vi "MemberAttendance Factory.vi"(8 "error in (no error)":errorcluster, 10 "2D Data":string[][](array[string]), 11 "ExcelReader in":refnum<class "ExcelReader.lvclass">) -> (0 "error out":errorcluster, 2 "MemberAttendance":refnum<class "MemberAttendance.lvclass">[](array[class]), 3 "ExcelReader out":refnum<class "ExcelReader.lvclass">)   [LabVIEW 2015, in "Admin_Actor.lvlib" / "ExcelReader.lvclass"]
uses:
  ExcelReader.lvclass
  MemberAttendance/MemberAttendance.lvclass
  g_variable/g_Excel Attributes.vi
  Database/Date_Excel/ExceelDate.lvclass
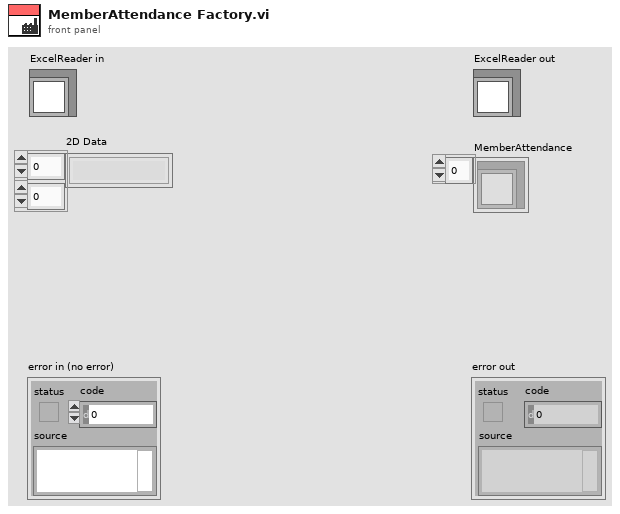
[diagram p1: front panel]
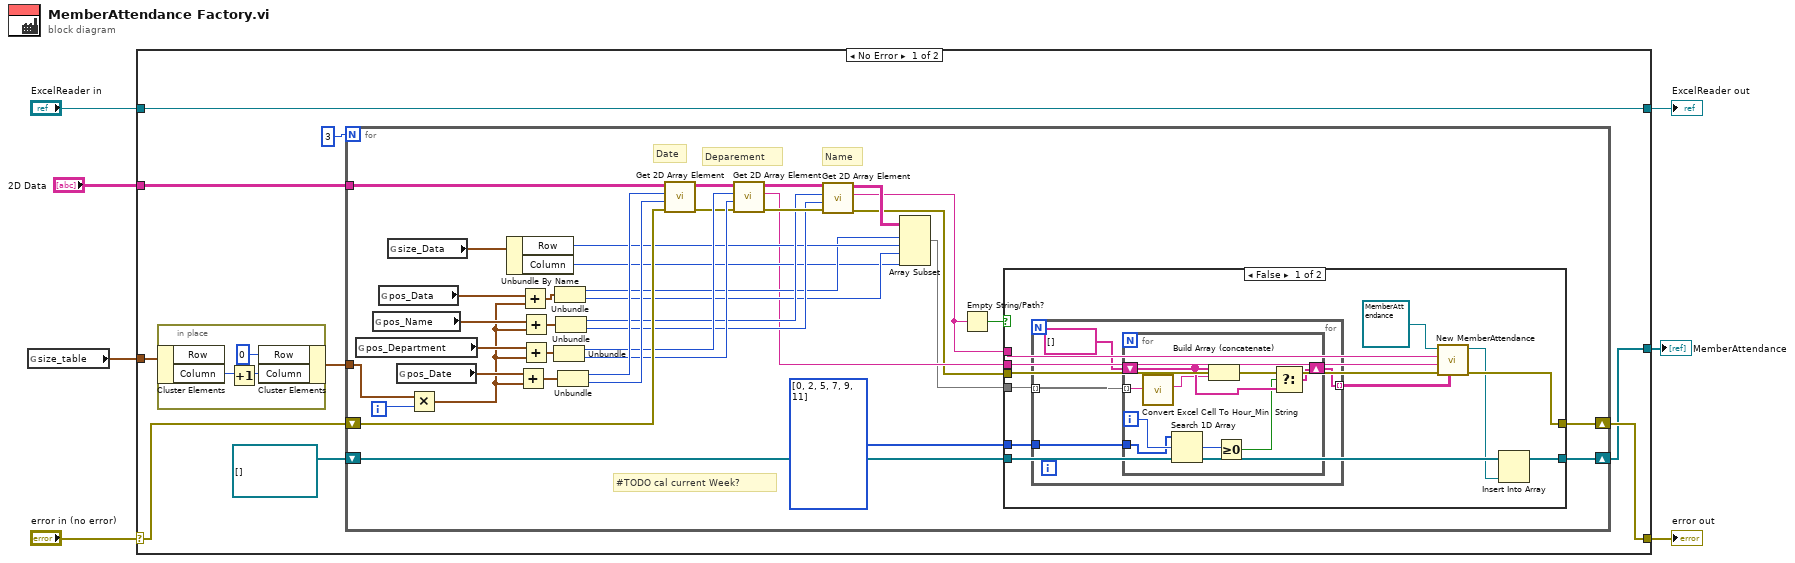
[diagram p0: block diagram]
diagram:
  n1 = global read "g_Excel Attributes.vi" "size_table"() -> (w2:cluster{"Row":i32, "Column":i32})
  n2 = case shown="No Error" "error in (no error)" {
    selector: "error in (no error)" -> [w13 w85]
    tunnel: [w12 w85] -> w6
    tunnel: [w16 w84] -> w4
    tunnel: "ExcelReader in" -> [w16 w84]
    tunnel: "2D Data" -> [w14 _]
    tunnel: w2 -> [w9 _]
    tunnel: [w10 _] -> w1
    frame No Error {
      n3 = in-place {
        n4 = in-place-cluster #1(w9) -> ("Column"=w19:i32)  [unwired: 1 out]
        n5 = Increment(x=w19) -> (x+1=w18:i32)
        n6 = in-place-cluster #1("Row"=0, "Column"=w18) -> (w8:cluster{"Row":i32, "Column":i32})
      }
      n7 = for {
        N: 3 -> [_]
        tunnel: w8 -> [w57]
        tunnel: w14 -> [w49]
        shift-right: [w25] -> w12
        shift-left: w13 -> [w51]
        shift-right: [w21] -> w10
        shift-left: refnum<class "MemberAttendance.lvclass">[] [] ("Array") -> [w24]
        i -> [w56]
        # "#TODO cal current Week?"
        # "Name"
        # "Deparement"
        # "Date"
        n8 = global read "g_Excel Attributes.vi" "pos_Department"() -> (w50:cluster{"Row":i32, "Column":i32})
        n9 = global read "g_Excel Attributes.vi" "pos_Name"() -> (w43:cluster{"Row":i32, "Column":i32})
        n10 = global read "g_Excel Attributes.vi" "pos_Data"() -> (w37:cluster{"Row":i32, "Column":i32})
        n11 = global read "g_Excel Attributes.vi" "size_Data"() -> (w34:cluster{"Row":i32, "Column":i32})
        n12 = global read "g_Excel Attributes.vi" "pos_Date"() -> (w55:cluster{"Row":i32, "Column":i32})
        n13 = Multiply(x=w57, y=w56) -> (x*y=w36:cluster{"Row":i32, "Column":i32})
        n14 = Unbundle By Name(w34) -> ("Row"=w33:i32, "Column"=w29:i32)
        n15 = Add(x=w55, y=w36) -> (x+y=w54:cluster{"Row":i32, "Column":i32})
        n16 = Add(x=w37, y=w36) -> (x+y=w32:cluster{"Row":i32, "Column":i32})
        n17 = Add(x=w43, y=w36) -> (x+y=w42:cluster{"Row":i32, "Column":i32})
        n18 = Add(x=w50, y=w36) -> (x+y=w44:cluster{"Row":i32, "Column":i32})
        n19 = Unbundle(w44) -> ("Row"=w47:i32, "Column"=w46:i32)
        n20 = Unbundle(w32) -> ("Row"=w31:i32, "Column"=w30:i32)
        n21 = Unbundle(w42) -> ("Row"=w39:i32, "Column"=w38:i32)
        n22 = Unbundle(w54) -> ("Row"=w53:i32, "Column"=w52:i32)
        n23 = call "Get 2D Array Element.vi"("error in (no error)"=w51, "Col"=w52, "Row"=w53, "Array"=w49) -> ("error out"=w45:errorcluster, "Array Out"=w48:string[][])  [unwired: 5 in, 1 out]
        n24 = call "Get 2D Array Element.vi"("error in (no error)"=w45, "Col"=w46, "Row"=w47, "Array"=w48) -> ("error out"=w41:errorcluster, "String"=w28:string, "Array Out"=w40:string[][])  [unwired: 5 in]
        n25 = call "Get 2D Array Element.vi"("error in (no error)"=w41, "Col"=w38, "Row"=w39, "Array"=w40) -> ("error out"=w26:errorcluster, "String"=w23:string, "Array Out"=w35:string[][])  [unwired: 5 in]
        n26 = Array Subset(array=w35, index (row)=w31, length (row)=w33, index (col)=w30, length (col)=w29) -> (w27:string[][])
        n27 = Empty String/Path?(string/path=w23) -> (empty?=w22:bool)
        n28 = case shown="False" w22 {
          tunnel: w23 -> [w67 _]
          tunnel: w28 -> [w66 _]
          tunnel: w27 -> [w60 _]
          tunnel: w26 -> [w65 w82]
          tunnel: [w64 w82] -> w25
          tunnel: [w61 w83] -> w21
          tunnel: w24 -> [w63 w83]
          tunnel: i32[] [0, 2, 5, 7, 9, 11] -> [w58 _]
          frame False {
            n29 = for {
              tunnel: w60 -> [w72] mode=indexing
              tunnel: [w70] -> w59 mode=indexing
              tunnel: w58 -> [w69]
              n30 = for {
                tunnel: w72 -> [w78] mode=indexing
                shift-right: [w79] -> w70
                shift-left: string[] [] -> [w80]
                tunnel: w69 -> [w75]
                i -> [w76]
                n31 = call "Convert Excel Cell To Hour_Min  String.vi"("Hour:Min(\"\")"=w78) -> ("Hour:Min(\"\")"=w77:string)  [unwired: 8 in, 2 out]
                n32 = Search 1D Array(1D array=w75, element=w76) -> (index of element=w74:i32)  [unwired: 1 in]
                n33 = Build Array (concatenate)(w80, w77) -> (w81:string[])
                n34 = Greater Or Equal To 0?(x=w74) -> (x >= 0?=w73:bool)
                n35 = Select(t=w81, s=w73, f=w80) -> (s? t:f=w79:string[])
              }
            }
            n36 = call "New MemberAttendance.vi"("AttendanceData"=w59, "error in (no error)"=w65, "Department(\"\")"=w66, "Name(\"\")"=w67, "MemberAttendance in"=refnum<class "MemberAttendance.lvclass"> refnum ("Admin_Actor.lvlib:MemberAttendance.lvclass")) -> ("error out"=w64:errorcluster, "MemberAttendance out"=w62:refnum<class "MemberAttendance.lvclass">)  [unwired: 5 in]
            n37 = Insert Into Array(array=w63, new element=w62) -> (w61:refnum<class "MemberAttendance.lvclass">[])  [unwired: 1 in]
          }
          frame True {
          }
        }
      }
    }
    frame Error {
    }
  }
  "error out" <- w6
  "ExcelReader out" <- w4
  "MemberAttendance" <- w1
